vi "DataVIS_Get_Cursor_Indices.vi"(8 "error in (no error)":errorcluster, 9 "Vslow":dbl[](array[numeric]), 10 "Vfast":dbl[][](array[numeric]), 11 "Cursor Graph":refnum<vi>) -> (0 "error out":errorcluster, 1 "Slow Indices":dbl[](array[numeric]), 2 "Slow Index (Cursor Y)":dbl, 3 "Fast Index (Cursor X) (IDK why it's an array)":dbl[](array[numeric]), 4 "Raw Cursor Position":T1, 5 "Fresh Y":bool, 7 "Fresh X":bool)   [LabVIEW 2016]
uses:
  <vilib>/Utility/miscctls.llb/LVPointDoubleTypeDef.ctl
  <vilib>/gmath/NI_Gmath.lvlib
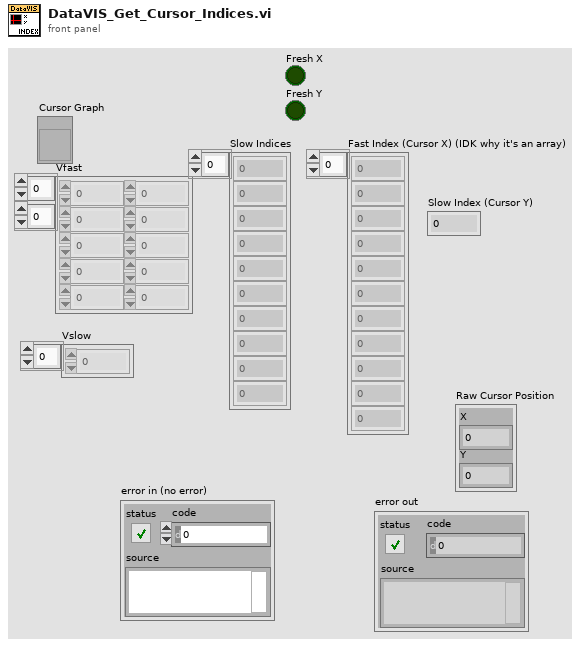
[diagram p1: front panel]
types:
  T1 = typedef "LVPointDoubleTypeDef.ctl" = cluster{"X":dbl, "Y":dbl}
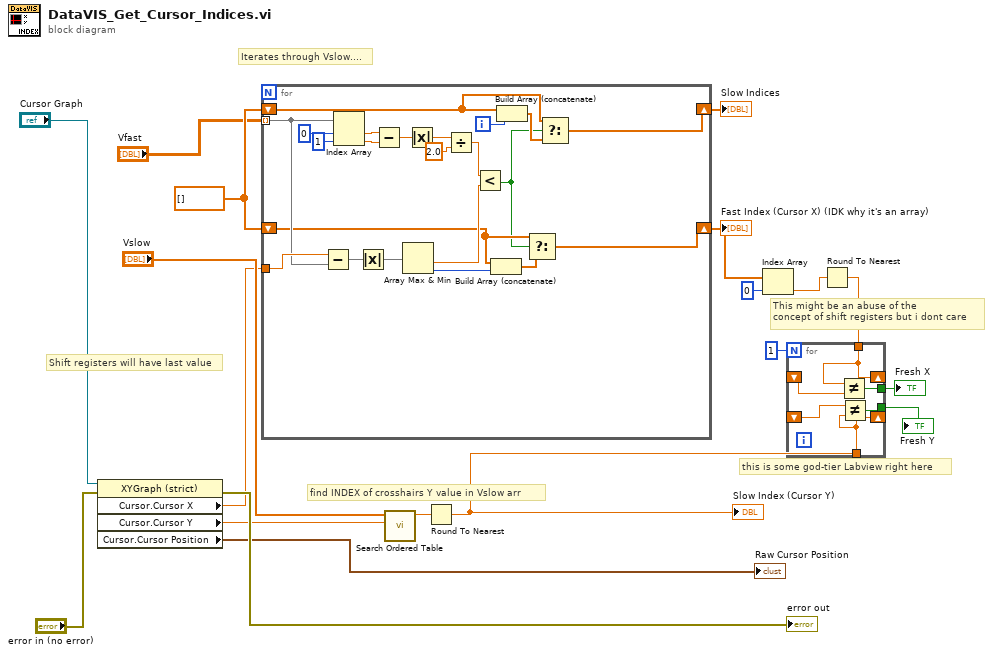
[diagram p0: block diagram]
diagram:
  w19 = dbl[] []
  # "this is some god-tier Labview right here"
  # "This might be an abuse of the \nconcept of shift registers but i dont care"
  # "Shift registers will have last value"
  # "Iterates through Vslow...."
  # "find INDEX of crosshairs Y value in Vslow arr"
  n1 = property class="XYGraph (strict)"(reference="Cursor Graph", error in="error in (no error)") -> (error out=→"error out":errorcluster, "Cursor.Cursor X"=w11:dbl, "Cursor.Cursor Y"=w10:dbl, "Cursor.Cursor Position"=→"Raw Cursor Position":T1)  [unwired: 1 out]
  n2 = for {
    tunnel: "Vfast" -> [w33] mode=indexing
    shift-right: [w21] -> w17
    shift-left: w19 -> [w23]
    shift-right: [w20] -> w7
    shift-left: w19 -> [w26]
    tunnel: w11 -> [w34]
    i -> [w25]
    n3 = Subtract(x=w34, y=w33) -> (x-y=w32:dbl[])
    n4 = Index Array(array=w33, index #1=0 ("index"), index #2=1 ("index")) -> (element #1=w39:dbl, element #2=w38:dbl)
    n5 = Absolute Value(x=w32) -> (abs(x)=w31:dbl[])
    n6 = Subtract(x=w39, y=w38) -> (x-y=w37:dbl)
    n7 = Array Max & Min(array=w31) -> (min value=w29:dbl, min index (indices)=w28:i32)  [unwired: 2 out]
    n8 = Absolute Value(x=w37) -> (abs(x)=w35:dbl)
    n9 = Divide(x=w35, y=2.0) -> (x/y=w30:dbl)
    n10 = Less?(x=w30, y=w29) -> (x < y?=w22:bool)
    n11 = Build Array (concatenate)(w26, w28) -> (w27:dbl[])
    n12 = Build Array (concatenate)(w23, w25) -> (w24:dbl[])
    n13 = Select(t=w26, s=w22, f=w27) -> (s? t:f=w20:dbl[])
    n14 = Select(t=w23, s=w22, f=w24) -> (s? t:f=w21:dbl[])
  }
  "Slow Indices" <- w17
  "Fast Index (Cursor X) (IDK why it's an array)" <- w7
  n15 = call <vilib>:"Search Ordered Table.vi"("x value"=w10, "ordered x array"="Vslow") -> ("fractional index"=w13:dbl)  [unwired: 9 in]
  n16 = Round To Nearest(number=w13) -> (nearest integer value=w5:dbl)
  "Slow Index (Cursor Y)" <- w5
  n17 = Index Array(array=w7, index=0) -> (element=w4:dbl)
  n18 = Round To Nearest(number=w4) -> (nearest integer value=w3:dbl)
  n19 = for {
    N: 1 -> [_]
    shift-right: [w47] -> _
    shift-left: _ -> [w46]
    shift-right: [w45] -> _
    shift-left: _ -> [w44]
    tunnel: w3 -> [w47]
    tunnel: w5 -> [w45]
    tunnel: [w43] -> w2
    tunnel: [w42] -> w1
    n20 = Not Equal?(x=w47, y=w46) -> (x != y?=w43:bool)
    n21 = Not Equal?(x=w44, y=w45) -> (x != y?=w42:bool)
  }
  "Fresh X" <- w2
  "Fresh Y" <- w1
